vi "TCF to Sequence Generator.vi"() -> ()   [LabVIEW 2018]
uses:
  Classes/niRFSTS Sequence Flow/niRFSTS Sequence Flow.lvclass
panel:
  in  "Prepend Measurement Result Names?":bool
  in  "Only include evaluations from test limits file?":bool
  in  "Generate":bool
  in  "stop":bool
  in  "Create Focus Calibration Definition File?":bool=TRUE
  in  "Use Existing Test Numbers and Transforms?":bool
  in  "Limits File Path":path
  out "Measurement Insertion Progress":u32(slide) caption="Initializing..." max=321 scale=0.0..321.0
  out "error out":errorcluster
  in  "Test Conditions File":path
  in  "New Sequence File Path":path
  in  "Template Path":path
  # "TCF to Sequence Generator"
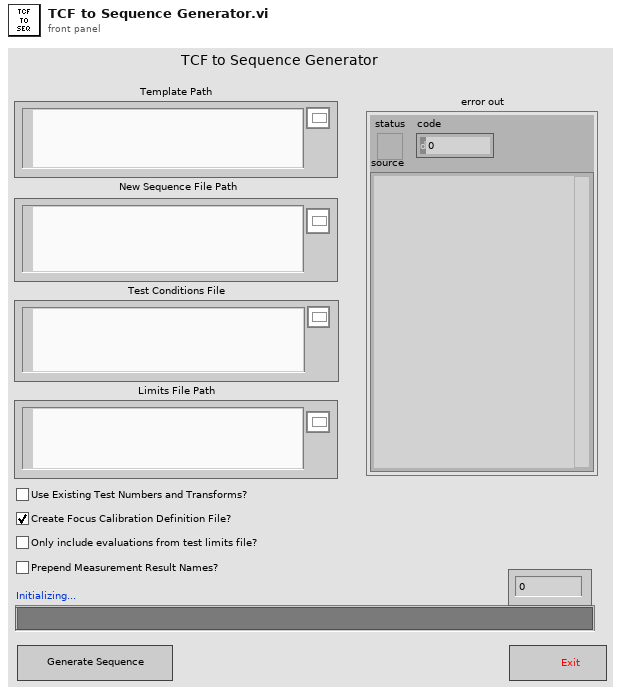
[diagram p1: front panel]
types:
  T1 = typedef "niRFSTS Sequence Flow.lvclass/Session Handle.ctl" = refnum<data-value>
  T2 = enum32{"invalid app kind", "Development System", "Run Time System", "Student Edition", "Embedded LabVIEW", "Evaluation", "Custom"}
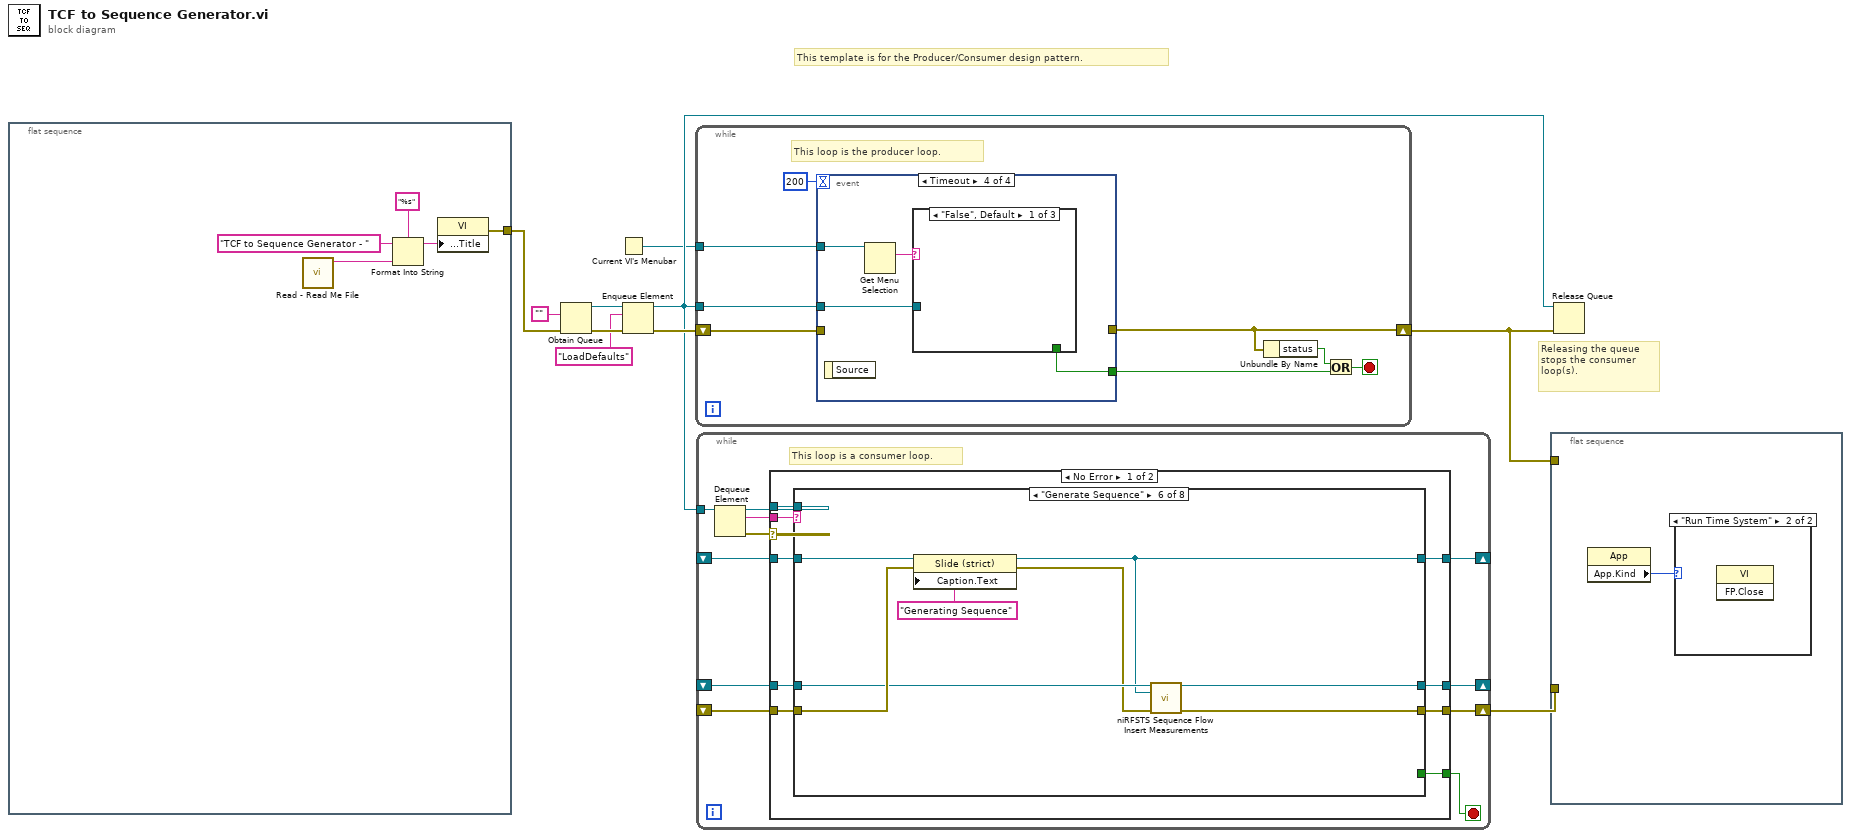
[diagram p0: block diagram]
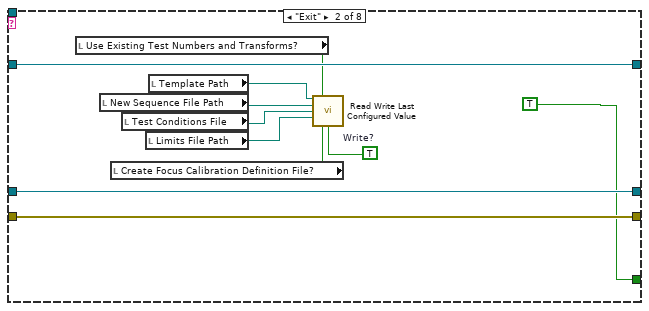
[diagram p4: hidden frame]
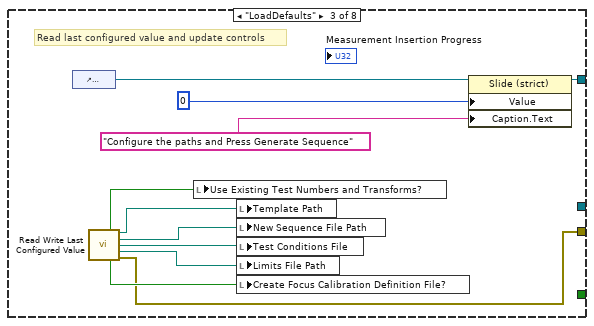
[diagram p5: hidden frame]
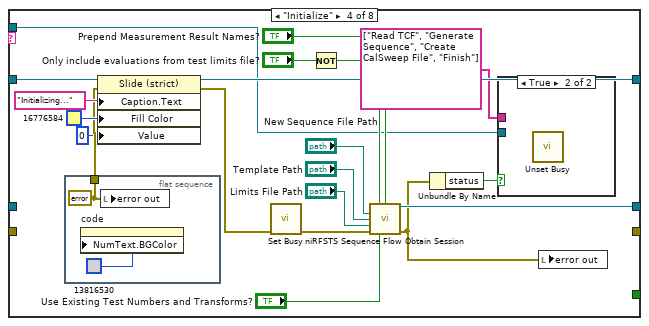
[diagram p6: hidden frame]
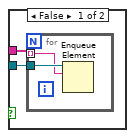
[diagram p7: hidden frame]
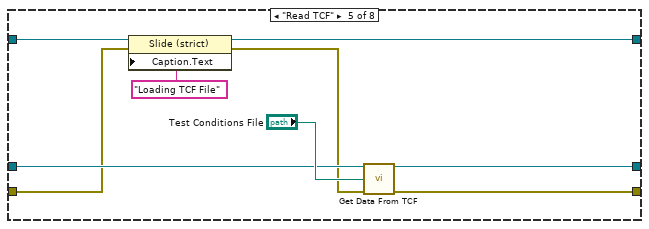
[diagram p8: hidden frame]
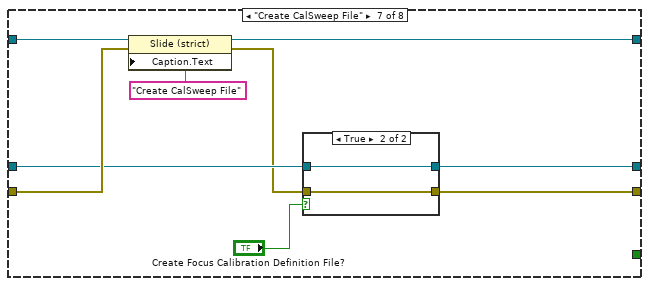
[diagram p9: hidden frame]
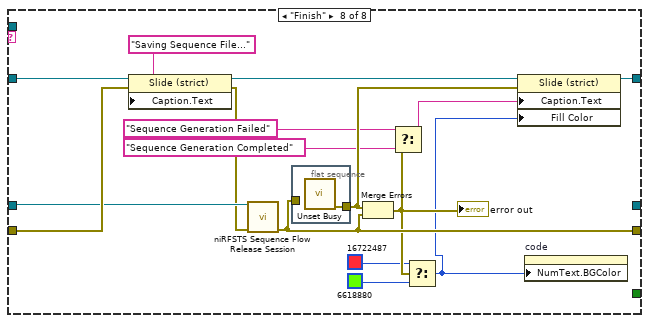
[diagram p11: hidden frame]
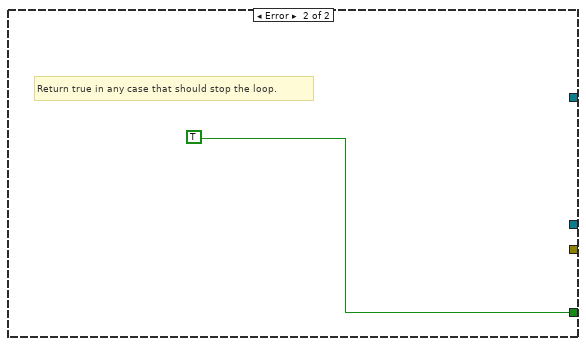
[diagram p12: hidden frame]
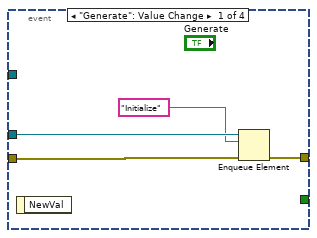
[diagram p13: hidden frame]
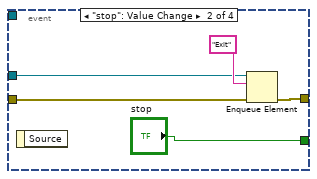
[diagram p14: hidden frame]
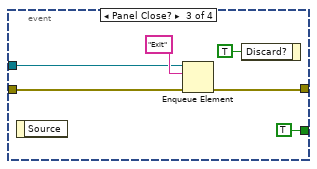
[diagram p15: hidden frame]
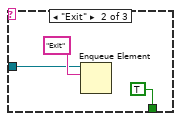
[diagram p16: hidden frame]
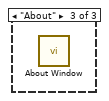
[diagram p17: hidden frame]
diagram:
  # "Releasing the queue stops the consumer loop(s)."
  # "This template is for the Producer/Consumer design pattern."
  n1 = flat-sequence {
    tunnel: [w12] -> w2
    frame #0 {
      n2 = call "Read - Read Me File.vi"() -> ("Version"=w11:string)  [unwired: 10 in, 1 out]
      n3 = Format Into String(format string="%s", initial string="TCF to Sequence Generator - " ("Front Panel Window:Title"), w11) -> (resulting string=w13:string)  [unwired: 1 in, 1 out]
      n4 = property class="VI"("Front Panel.Title"=w13) -> (error out=w12:errorcluster)  [unwired: 2 in, 1 out]
    }
  }
  n5 = Obtain Queue(element data type="" ("data (can be any type)"), error in (no error)=w2) -> (queue out=w7:refnum<queue>, error out=w9:errorcluster)  [unwired: 3 in, 1 out]
  n6 = Current VI's Menubar() -> (w1:refnum<k9>)
  n7 = Enqueue Element(queue=w7, element="LoadDefaults" ("data (can be any type)"), error in (no error)=w9) -> (queue out=w6:refnum<queue>, error out=w8:errorcluster)  [unwired: 1 in, 1 out]
  n8 = while {
    shift-right: [w19] -> w3
    shift-left: w8 -> [w22]
    tunnel: w6 -> [w23]
    tunnel: w1 -> [w16]
    stop <- w20 stop-if-true
    # "This loop is the producer loop."
    n9 = event shown="[3] Timeout" {
      selector: _ -> [_ _ _ _]
      dyn-events: _ -> [_ _ _ _]
      timeout: 200 -> [_ _ _ _]
      tunnel: w23 -> [w27 w28 w36 w41]
      tunnel: w22 -> [w26 w30 w37 _]
      tunnel: [w25 w29 w34 _] -> w19
      tunnel: [_ "stop" TRUE ("stop") w39] -> w21
      tunnel: w16 -> [_ _ _ w42]
      event "Generate": Value Change {
        n10 = event-data() -> ()  [unwired: 1 in, 1 out]
        n11 = Enqueue Element(queue=w27, element="Initialize", error in (no error)=w26) -> (error out=w25:errorcluster)  [unwired: 1 in, 2 out]
      }
      event "stop": Value Change {
        n12 = event-data() -> ()  [unwired: 1 in, 1 out]
        n13 = Enqueue Element(queue=w28, element="Exit", error in (no error)=w30) -> (error out=w29:errorcluster)  [unwired: 1 in, 2 out]
      }
      event Panel Close? {
        n14 = event-data() -> ()  [unwired: 1 in, 1 out]
        n15 = Enqueue Element(queue=w36, element="Exit", error in (no error)=w37) -> (error out=w34:errorcluster)  [unwired: 1 in, 2 out]
        n16 = event-data("Discard?"=TRUE) -> ()  [unwired: 1 in, 1 out]
      }
      event Timeout {
        n17 = event-data() -> ()  [unwired: 1 in, 1 out]
        n18 = Get Menu Selection(0:w42) -> (6:w40:string)  [unwired: 3 in, 4 out]
        n19 = case shown="\"False\", Default" w40 {
          tunnel: w41 -> [_ w44 _]
          tunnel: [_ TRUE ("stop") _] -> w39
          frame "False", Default {
          }
          frame "Exit" {
            n20 = Enqueue Element(queue=w44, element="Exit") -> ()  [unwired: 2 in, 3 out]
          }
          frame "About" {
            n21 = call "About Window.vi"() -> ()  [unwired: 12 in]
          }
        }
      }
    }
    n22 = Unbundle By Name(w19) -> ("status"=w18:bool)
    n23 = Or(x=w18, y=w21) -> (x .or. y?=w20:bool)
  }
  n24 = while {
    tunnel: w6 -> [w56]
    shift-right: [w52] -> w4
    shift-left: _ -> [w48]
    shift-right: [w51] -> _
    shift-left: _ -> [w50]
    shift-right: [w49] -> _
    shift-left: _ -> [w47]
    stop <- w53 stop-if-true
    # "This loop is a consumer loop."
    n25 = Dequeue Element(queue=w56) -> (queue out=w46:refnum<queue>, element=w54:string, error out=w55:errorcluster)  [unwired: 2 in, 1 out]
    n26 = case shown="No Error" w55 {
      tunnel: w54 -> [w65 _]
      tunnel: [w58 TRUE] -> w53
      tunnel: [w64 _] -> w52
      tunnel: [w63 _] -> w51
      tunnel: w50 -> [w62 _]
      tunnel: [w61 _] -> w49
      tunnel: w48 -> [w60 _]
      tunnel: w47 -> [w59 _]
      tunnel: w46 -> [w57 _]
      frame No Error {
        n27 = case shown="\"Generate Sequence\"" w65 {
          tunnel: [w66 w77 w80 _ w122 w128 w135 w158] -> w64
          tunnel: [w68 w79 w88 w104 w120 w127 w140 w155] -> w63
          tunnel: w62 -> [w68 w79 _ w105 w121 w133 w142 w162]
          tunnel: [w67 w78 _ w102 w123 w130 w137 _] -> w61
          tunnel: w60 -> [w66 w77 _ _ w119 w132 w141 w161]
          tunnel: w59 -> [w67 w78 _ _ w124 w131 w138 w160]
          tunnel: [_ TRUE _ _ _ _ _ _] -> w58
          tunnel: w57 -> [_ _ _ w93 _ _ _ _]
          frame Default {
          }
          frame "Exit" {
            w69 = TRUE  # Write?
            n28 = local read "Use Existing Test Numbers and Transforms?"() -> (w70:bool)
            n29 = local read "New Sequence File Path"() -> (w74:path)
            n30 = local read "Create Focus Calibration Definition File?"() -> (w71:bool)
            n31 = local read "Test Conditions File"() -> (w73:path)
            n32 = local read "Limits File Path"() -> (w72:path)
            n33 = local read "Template Path"() -> (w75:path)
            n34 = call "Read Write Last Configured Value.vi"("Template Sequence Path"=w75, "Use Existing Test Numbers?"=w70, "New Sequence File Path"=w74, "Test Conditions File"=w73, "Limits File Path"=w72, "Create Focus Calibration Definition File?"=w71, "Write?"=w69) -> ()  [unwired: 2 in, 7 out]
          }
          frame "LoadDefaults" {
            # "Read last configured value and update controls"
            n35 = control-ref of="Measurement Insertion Progress"() -> (w90:refnum<vi>)
            n36 = call "Read Write Last Configured Value.vi"() -> ("Use Existing Test Numbers? 2"=w86:bool, "Template Sequence"=w85:path, "New Sequence File"=w84:path, "Test Conditions File"=w83:path, "Limits File"=w82:path, "Create Focus Calibration Definition File? 2"=w81:bool, "error out"=w80:errorcluster)  [unwired: 9 in]
            n37 = local write "Use Existing Test Numbers and Transforms?"(w86) -> ()
            n38 = local write "Template Path"(w85) -> ()
            n39 = local write "New Sequence File Path"(w84) -> ()
            n40 = local write "Test Conditions File"(w83) -> ()
            n41 = local write "Limits File Path"(w82) -> ()
            n42 = local write "Create Focus Calibration Definition File?"(w81) -> ()
            n43 = property class="Slide (strict)"(reference=w90, "Value"=u32 0, "Caption.Text"="Configure the paths and Press Generate Sequence") -> (reference out=w88:refnum<vi>)  [unwired: 1 in, 1 out]
          }
          frame "Initialize" {
            n44 = flat-sequence {
              tunnel: [w116] -> w99
              frame #0 {
                w116 = errorcluster {"status"=FALSE, "code"=0, "source"=""} ("error out")
                n45 = property on="code" class="DigNum (strict)"("NumText.BGColor"=u32 13816530 ("Color Box")) -> ()  [unwired: 2 in, 2 out]
                n46 = local write "error out"(w116) -> ()
              }
            }
            n47 = property class="Slide (strict)"(reference=w105, error in=w99, "Caption.Text"="Initializing...", "Fill Color"=u32 16776584 ("Color Box"), "Value"=u32 0) -> (reference out=w104:refnum<vi>, error out=w103:errorcluster)
            n48 = call <vilib>:"Set Busy.vi"("error in (no error)"=w103) -> ("error out"=w110:errorcluster)  [unwired: 9 in, 1 out]
            n49 = Not(x="Only include evaluations from test limits file?") -> (.not. x?=w96:bool)
            n50 = call "niRFSTS Sequence Flow Obtain Session.vi"("Include All Evaluations?"=w96, "Prepend Result Names?"="Prepend Measurement Result Names?", "New Sequence File Path"="New Sequence File Path", "Template Path"="Template Path", "Limits File Path"="Limits File Path", "error in (no error)"=w110, "Use Existing Test Numbers?"="Use Existing Test Numbers and Transforms?") -> ("Session Handle"=w102:T1, "error out"=w94:errorcluster)  [unwired: 7 in]
            n51 = Unbundle By Name(w94) -> ("status"=w91:bool)
            n52 = case shown="True" w91 {
              tunnel: w93 -> [w112 _]
              tunnel: string[] ["Read TCF", "Generate Sequence", "Create CalSweep File", "Finish"] -> [w111 _]
              frame False {
                n53 = for {
                  tunnel: w112 -> [w114]
                  tunnel: w111 -> [w113] mode=indexing
                  n54 = Enqueue Element(queue=w114, element=w113) -> ()  [unwired: 2 in, 3 out]
                }
              }
              frame True {
                n55 = call <vilib>:"Unset Busy.vi"() -> ()  [unwired: 11 in, 1 out]
              }
            }
            n56 = local write "error out"(w94) -> ()
          }
          frame "Read TCF" {
            n57 = property class="Slide (strict)"(reference=w121, error in=w119, "Caption.Text"="Loading TCF File") -> (reference out=w120:refnum<vi>, error out=w118:errorcluster)
            n58 = call "Get Data From TCF.vi"("Session Handle in"=w124, "Test Conditions File"="Test Conditions File", "error in (no error)"=w118) -> ("Session Handle out"=w123:T1, "error out"=w122:errorcluster)  [unwired: 11 in]
          }
          frame "Generate Sequence" {
            n59 = property class="Slide (strict)"(reference=w133, error in=w132, "Caption.Text"="Generating Sequence") -> (reference out=w127:refnum<vi>, error out=w129:errorcluster)
            n60 = call "niRFSTS Sequence Flow Insert Measurements.vi"("Session Handle in"=w131, "Measurement Insertion Progress"=w127, "error in (no error)"=w129) -> ("Session Handle out"=w130:T1, "error out"=w128:errorcluster)  [unwired: 11 in]
          }
          frame "Create CalSweep File" {
            n61 = property class="Slide (strict)"(reference=w142, error in=w141, "Caption.Text"="Create CalSweep File") -> (reference out=w140:refnum<vi>, error out=w136:errorcluster)
            n62 = case shown="True" "Create Focus Calibration Definition File?" {
              tunnel: w138 -> [w144 w146]
              tunnel: [w144 w146] -> w137
              tunnel: w136 -> [w143 w145]
              tunnel: [w143 w145] -> w135
              frame False {
              }
              frame True {
              }
            }
          }
          frame "Finish" {
            n63 = property class="Slide (strict)"(reference=w162, error in=w161, "Caption.Text"="Saving Sequence File...") -> (reference out=w156:refnum<vi>, error out=w159:errorcluster)
            n64 = call "niRFSTS Sequence Flow Release Session.vi"("Session Handle"=w160, "error in (no error)"=w159) -> ("error out"=w158:errorcluster)  [unwired: 13 in]
            n65 = flat-sequence {
              tunnel: [w163] -> w154
              tunnel: w158 -> [_]
              frame #0 {
                n66 = call <vilib>:"Unset Busy.vi"() -> ("error out"=w163:errorcluster)  [unwired: 11 in]
              }
            }
            n67 = Merge Errors(w154, w158) -> (w149:errorcluster)
            "error out" <- w149
            n68 = Select(t="Sequence Generation Failed" ("Caption.Text"), s=w149, f="Sequence Generation Completed" ("Caption.Text")) -> (s? t:f=w151:string)
            n69 = Select(t=u32 16722487 ("Color Box"), s=w149, f=u32 6618880 ("Color Box")) -> (s? t:f=w147:u32)
            n70 = property class="Slide (strict)"(reference=w156, error in=w154, "Caption.Text"=w151, "Fill Color"=w147) -> (reference out=w155:refnum<vi>)  [unwired: 1 out]
            n71 = property on="code" class="DigNum (strict)"("NumText.BGColor"=w147) -> ()  [unwired: 2 in, 2 out]
          }
        }
      }
      frame Error {
        # "Return true in any case that should stop the loop."
      }
    }
  }
  n72 = flat-sequence {
    tunnel: w4 -> [_]
    tunnel: w3 -> [_]
    frame #0 {
      n73 = property class="App"() -> ("App.Kind"=w165:T2)  [unwired: 2 in, 2 out]
      n74 = case shown="\"Run Time System\"" w165 {
        frame "invalid app kind", Default {
        }
        frame "Run Time System" {
          n75 = invoke class="VI" method="FP.Close"() -> ()  [unwired: 3 in, 3 out]
        }
      }
    }
  }
  n76 = Release Queue(queue=w6, error in (no error)=w3) -> ()  [unwired: 1 in, 3 out]
